vi "Jaguar Status.vi"(3 "Enable":bool) -> ()   [LabVIEW 2011]
uses:
  <vilib>/Rock Robotics/WPI/CAN/Jaguar/SubVIs/WPI_CANJaguar_ControlMode.ctl
  <vilib>/Rock Robotics/WPI/CAN/Jaguar/SubVIs/WPI_CANJaguar_StatusSelect.ctl
panel:
  out "I":dbl
  out "D":dbl
  out "P":dbl
  out "Control Mode":T1
  in  "Motor Name":string(combo)="Front Left Drive"
  out "Comm Fault":bool caption="Boolean"
  out "Gate Driver Fault":bool caption="Boolean"
  out "Bus Voltage Fault":bool caption="Boolean"
  out "Temperature Fault":bool caption="Boolean"
  out "Current Fault":bool caption="Boolean"
  out "Power Cycle":bool caption="Boolean"
  in  "Clear":bool
  # "Jaguar Status"
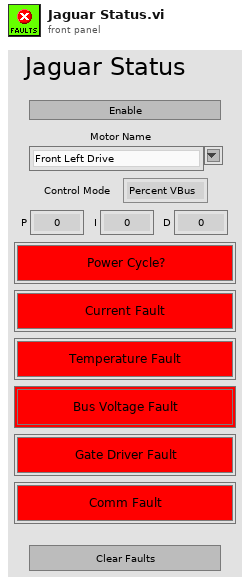
[diagram p1: front panel]
types:
  T1 = typedef "WPI_CANJaguar_ControlMode.ctl" = enum8{"Percent VBus", "Current", "Speed", "Position", "Voltage"}
  T2 = typedef "WPI_CANJaguar_StatusSelect.ctl" = enum16{"Output Percent VBus", "Output Voltage", "Bus Voltage", "Current", "Temperature", "Position", "Speed", "Limit Switches", "Faults", "Fault Counters", "Power Cycle"}
  T3 = typedef "WPI_MotorControlDeviceRef.ctl" = cluster{"DeviceStatus":errorcluster, "Type":enum16{"PWM", "CAN"}, "PWM":cluster{"Digital Module":T4, "PWM Channel":T5, "DeadBand":T6}, "CAN":cluster{"Device Number":u8, "Control Mode":T1, "Semaphore":T7, "Max Vout":dbl}, "Invert":bool, "TransformRef":T8, "InvTransformRef":T8}
  T4 = typedef "FPGA_TypedefDigitalModule.ctl" = enum16{"Digital Module 1", "Digital Module 2"}
  T5 = typedef "FPGA_DIOPWMChannel.ctl" = enum8{"PWM 1", "PWM 2", "PWM 3", "PWM 4", "PWM 5", "PWM 6", "PWM 7", "PWM 8", "PWM 9", "PWM 10", "Invalid"}
  T6 = typedef "WPI_PWMDeadband.ctl" = cluster{"Name":string, "maxPositivePwm":i32, "minPositivePwm":i32, "centerPwm":i32, "maxNegativePwm":i32, "minNegativePwm":i32, "angularRange":u16}
  T7 = typedef "Semaphore RefNum" = refnum<k1>
  T8 = typedef "WPI_PWMTransform_ConPane.ctl" = refnum<vi>
  T9 = typedef "WPI_CANJaguar_Status.ctl" = cluster{"Output Percent VBus":dbl, "Output Voltage":dbl, "Bus Voltage":dbl, "Current":dbl, "Temperature":dbl, "Position":dbl, "Speed":dbl, "Limits":cluster{"Forward Limit":bool, "Reverse Limit":bool, "Forward Soft Limit":bool, "Reverse Soft Limit":bool, "Sticky Forward Limit":bool, "Sticky Reverse Limit":bool, "Sticky Forward Soft Limit":bool, "Sticky Reverse Soft Limit":bool}, "Faults":cluster{"Current Fault":bool, "Temperature Fault":bool, "Bus Voltage Fault":bool, "Gate Driver Fault":bool, "Comm Fault":bool}, "Fault Counters":cluster{"Current Faults":u8, "Temperature Faults":u8, "Bus Voltage Faults":u8, "Gate Driver Faults":u8, "Comm Faults":u8, "CAN Status":u8, "CAN RX Errors":u8, "CAN TX Errors":u8}, "Power Cycle":bool}
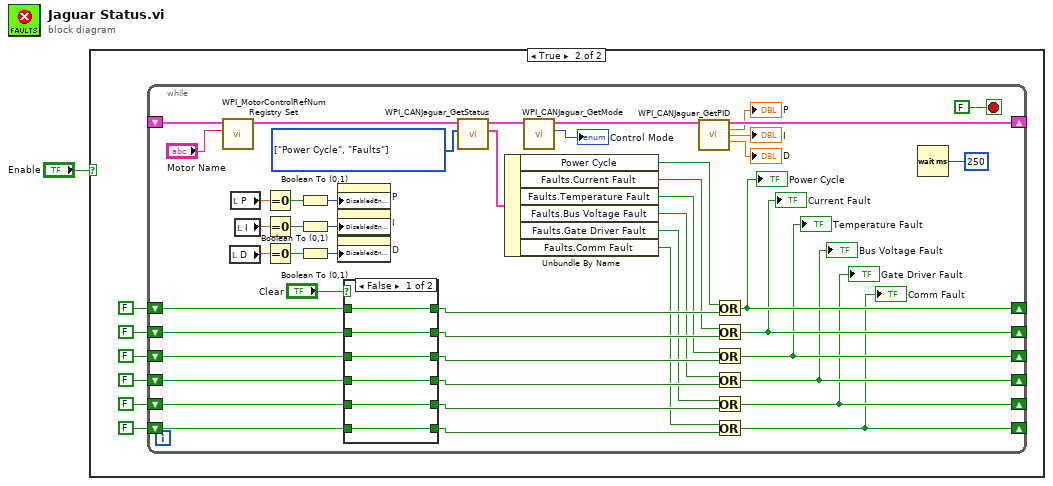
[diagram p0: block diagram]
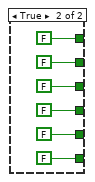
[diagram p3: hidden frame]
diagram:
  n1 = case shown="True" "Enable" {
    frame False {
    }
    frame True {
      n2 = while {
        shift-right: [w26] -> _
        shift-left: _ -> [w50]
        shift-right: [w36] -> _
        shift-left: FALSE -> [w47]
        shift-right: [w35] -> _
        shift-left: FALSE -> [w46]
        shift-right: [w34] -> _
        shift-left: FALSE -> [w45]
        shift-right: [w33] -> _
        shift-left: FALSE -> [w44]
        shift-right: [w32] -> _
        shift-left: FALSE -> [w43]
        shift-right: [w31] -> _
        shift-left: FALSE -> [w42]
        stop <- FALSE stop-if-true
        w55 = T2[] [enum."Power Cycle", enum."Faults"] items=["Output Percent VBus", "Output Voltage", "Bus Voltage", "Current", "Temperature", "Position", "Speed", "Limit Switches", "Faults", "Fault Counters", "Power Cycle"] ("Status Select")
        n3 = call <vilib>:"WPI_MotorControlRefNum Registry Set.vi"("refnum name"="Motor Name", "MotorControlDevRef"=w50) -> ("MotorControlDevRef"=w51:T3)  [unwired: 8 in, 1 out]
        n4 = local read "D"() -> (w19:dbl)
        n5 = local read "P"() -> (w21:dbl)
        n6 = local read "I"() -> (w20:dbl)
        n7 = Equal To 0?(x=w21) -> (x = 0?=w18:bool)
        n8 = Equal To 0?(x=w20) -> (x = 0?=w16:bool)
        n9 = Equal To 0?(x=w19) -> (x = 0?=w15:bool)
        n10 = Boolean To (0,1)(Boolean=w18) -> (0, 1=w17:i16)
        n11 = Boolean To (0,1)(Boolean=w16) -> (0, 1=w14:i16)
        n12 = Boolean To (0,1)(Boolean=w15) -> (0, 1=w13:i16)
        n13 = property on="P" class="DigNum (strict)"("DisabledEnum"=w17) -> ()  [unwired: 2 in, 2 out]
        n14 = property on="I" class="DigNum (strict)"("DisabledEnum"=w14) -> ()  [unwired: 2 in, 2 out]
        n15 = property on="D" class="DigNum (strict)"("DisabledEnum"=w13) -> ()  [unwired: 2 in, 2 out]
        n16 = case shown="False" "Clear" {
          tunnel: [w61 FALSE] -> w48
          tunnel: w47 -> [w61 _]
          tunnel: w46 -> [w60 _]
          tunnel: w45 -> [w59 _]
          tunnel: w44 -> [w58 _]
          tunnel: w43 -> [w57 _]
          tunnel: w42 -> [w56 _]
          tunnel: [w60 FALSE] -> w41
          tunnel: [w59 FALSE] -> w40
          tunnel: [w58 FALSE] -> w39
          tunnel: [w57 FALSE] -> w38
          tunnel: [w56 FALSE] -> w37
          frame False {
          }
          frame True {
          }
        }
        n17 = call <vilib>:"WPI_CANJaguar_GetStatus.vi"("Status Select"=w55, "CAN Jaguar Ref"=w51) -> ("Status"=w54:T9, "CAN Jaguar Ref Out"=w28:T3)  [unwired: 7 in, 1 out]
        n18 = Unbundle By Name(w54) -> ("Power Cycle"=w52:bool, "Faults.Current Fault"=w12:bool, "Faults.Temperature Fault"=w11:bool, "Faults.Bus Voltage Fault"=w10:bool, "Faults.Gate Driver Fault"=w9:bool, "Faults.Comm Fault"=w8:bool)
        n19 = call <vilib>:"WPI_CANJaguar_GetMode.vi"("CAN Jaguar Ref"=w28) -> ("Control Mode"=→"Control Mode":T1, "CAN Jaguar Ref Out"=w27:T3)  [unwired: 8 in, 1 out]
        n20 = call <vilib>:"WPI_CANJaguar_GetPID.vi"("CAN Jaguar Ref"=w27) -> ("CAN Jaguar Ref Out"=w26:T3, "P"=→"P":dbl, "I"=→"I":dbl, "D"=→"D":dbl)  [unwired: 10 in, 1 out]
        n21 = Or(x=w52, y=w48) -> (x .or. y?=w36:bool)
        "Power Cycle" <- w36
        n22 = Or(x=w12, y=w41) -> (x .or. y?=w35:bool)
        "Current Fault" <- w35
        n23 = Or(x=w11, y=w40) -> (x .or. y?=w34:bool)
        "Temperature Fault" <- w34
        n24 = Or(x=w10, y=w39) -> (x .or. y?=w33:bool)
        "Bus Voltage Fault" <- w33
        n25 = Or(x=w9, y=w38) -> (x .or. y?=w32:bool)
        "Gate Driver Fault" <- w32
        n26 = Or(x=w8, y=w37) -> (x .or. y?=w31:bool)
        "Comm Fault" <- w31
        n27 = Wait (ms)(milliseconds to wait=u32 250) -> ()  [unwired: 1 out]
      }
    }
  }
